vi "Force Measurement.vi"() -> ()   [LabVIEW 2017]
uses:
  Pico Temperature.vi
panel:
  out "Balance Temperature":dbl(graph)
  out "Fx":dbl(graph)
  out "Start time":timestamp
  out "Output":string
  in  "Stop Button":bool
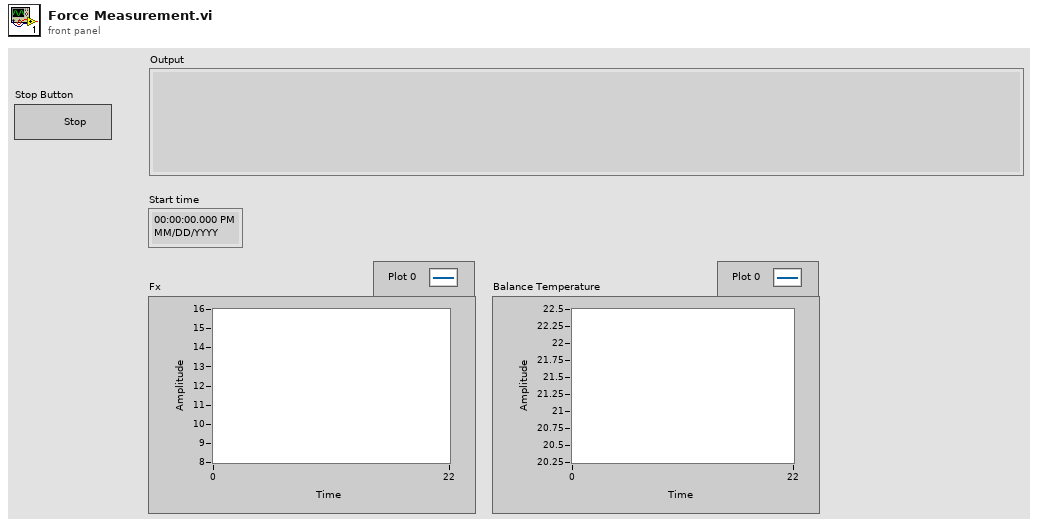
[diagram p1: front panel]
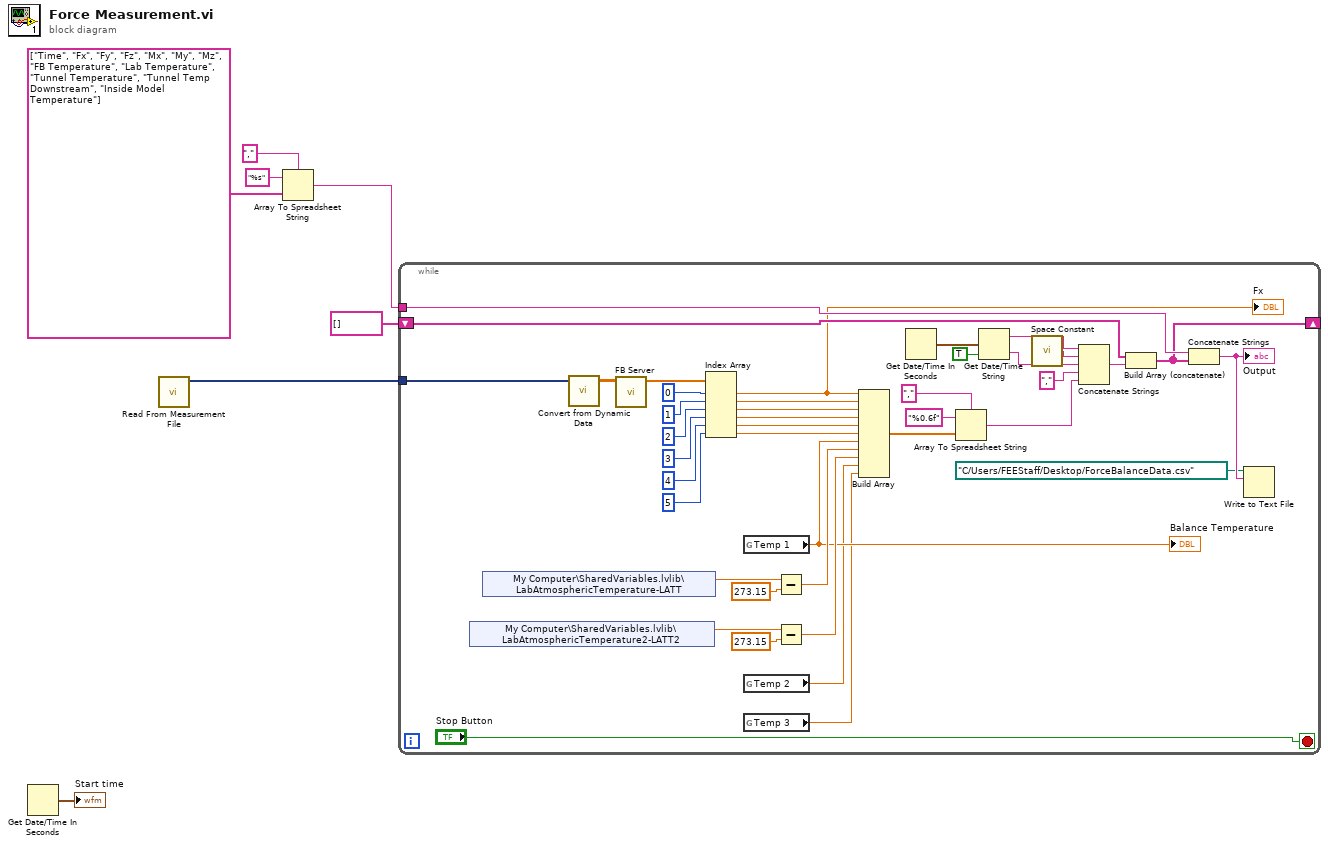
[diagram p0: block diagram]
diagram:
  n1 = Get Date/Time In Seconds() -> (seconds since 1Jan1904=→"Start time":timestamp)
  n2 = call "Read From Measurement File"() -> ("Signals"=w1:dynamicdata)  [unwired: 6 in, 5 out]
  n3 = Array To Spreadsheet String(delimiter (Tab)=",", array=string[] ["Time", "Fx", "Fy", "Fz", "Mx", "My", "Mz", "FB Temperature", "Lab Temperature", "Tunnel Temperature", "Tunnel Temp Downstream", "Inside Model Temperature"], 3:"%s" ("delimiter (Tab)")) -> (spreadsheet string=w3:string)
  n4 = while {
    shift-right: [w37] -> _
    shift-left: string[] [] -> [w39]
    tunnel: w3 -> [w38]
    tunnel: w1 -> [w20]
    stop <- "Stop Button" stop-if-true
    n5 = shared-variable "My Computer\\SharedVariables.lvlib\\LabAtmosphericTemperature2-LATT2"() -> (w19:dbl)  [unwired: 1 in, 1 out]
    n6 = shared-variable "My Computer\\SharedVariables.lvlib\\LabAtmosphericTemperature-LATT"() -> (w16:dbl)  [unwired: 1 in, 1 out]
    n7 = call "Convert from Dynamic Data"("Dynamic Data Type"=w20) -> ("Array"=w12:dbl[][])  [unwired: 3 in]
    n8 = call "FB Server.vi"("C2O"=w12) -> ("Fx                     Fy                     Fz                    Mx                   My                    Mz"=w33:dbl[])  [unwired: 9 in]
    n9 = Index Array(array=w33, index #1=0 ("disabled index (col)"), index #2=1 ("index (col)"), index #3=2 ("index (col)"), index #4=3 ("index (col)"), index #5=4 ("index (col)"), index #6=5 ("index (col)")) -> (element #1=w26:dbl, element #2=w25:dbl, element #3=w24:dbl, element #4=w23:dbl, element #5=w22:dbl, element #6=w21:dbl)
    "Fx" <- w26
    n10 = global read "Pico Temperature.vi" "Temp 1"() -> (w13:dbl)
    "Balance Temperature" <- w13
    n11 = global read "Pico Temperature.vi" "Temp 2"() -> (w9:dbl)
    n12 = global read "Pico Temperature.vi" "Temp 3"() -> (w8:dbl)
    n13 = Subtract(x=w16, y=273.15) -> (x-y=w15:dbl)
    n14 = Subtract(x=w19, y=273.15) -> (x-y=w14:dbl)
    n15 = Build Array(w26, w25, w24, w23, w22, w21, w13, w15, w14, w9, w8) -> (w36:dbl[])
    n16 = Get Date/Time In Seconds() -> (seconds since 1Jan1904=w45:timestamp)
    n17 = Array To Spreadsheet String(delimiter (Tab)=",", array=w36, 3:"%0.6f" ("format string")) -> (spreadsheet string=w41:string)
    n18 = Get Date/Time String(seconds (now)=w45, want seconds? (F)=TRUE) -> (date string=w11:string, time string=w43:string)  [unwired: 1 in]
    n19 = call <vilib>:"Space Constant.vi"() -> ("String"=w10:string)
    n20 = Concatenate Strings(w11, w10, w43, "," ("string"), w41) -> (w40:string)
    n21 = Build Array (concatenate)(w39, w40) -> (w37:string[])
    n22 = Concatenate Strings(w38, w37) -> (w35:string)
    "Output" <- w35
    n23 = Write to Text File(file (use dialog)=path "C:/Users/FEEStaff/Desktop/ForceBalanceData.csv", text=w35) -> ()  [unwired: 2 in, 3 out]
  }
